vi "ATE_Bandwidth_2.vi"() -> ()   [LabVIEW 2009]
doc: "RVP8 bandwidth measuring vi - reads the primary frequency of SPOL from the ATE_settings.txt file"
uses:
  Rvp8PowerData.ctl
  <vilib>/Analysis/NI_AALBase.lvlib
  <vilib>/Analysis/NI_AALPro.lvlib
panel:
  in  "Ready":bool
  out "Instructions":string="rvp8 bandwidth measuring vi\n\nBasic operation\n1 - configure ATE switches with the yellow 'Bandwidth Setup' button\n2 - measure the bandwidth with the red 'Calibrate' button\n3 - exit the program with the red 'Exit' button\n\nHints:\nWait for the green 'READY' light before clicking buttons\nClick blue buttons after making changes on 'Controls' tab\nCheck status tab before calibration"
  out "Real Time XY":cluster{dbl[], dbl[]}(graph)
  in  "Configuration 1":bool
  out "Cal Output File":path
  out "?":cluster{dbl[], dbl[]}[](graph)
  out "RVP8 Bandwidth":cluster{dbl[], dbl[]}[](graph)
  in  "DataSource":bool
  out "File Name":string
  in  "Data Directory":string="/home/operator/ate/data/rvp8_bw"
  in  "Set SigGen":bool
  in  "Initialize":bool
  in  "70 dB":bool
  in  "121 dB":bool
  in  "Switches":bool
  in  "Calibrate":bool
  in  "Stop":bool
  in  "ATE TABS":enum32{"Status", "Controls"}(tab)=enum."Controls"
  out "ATE Switch Status":T1
  out "121dB\nAttenuators":bool[](array[boolean])
  out "70dB\nAttenuators":bool[](array[boolean])
  out "RVP8 Power":T2 {"time" format="%<%H:%M:%S\n%Y/%m/%d>T"}
  out "Signal Generator Status":T3={"Freq (GHz)"=0.0, "RF Power (dBm)"=0.0, "RF Power"=TRUE} {"Freq (GHz)" format="%.5g"; "RF Power (dBm)" format="%.2g"}
  out "121 Verified":bool
  out "70 Verfied":bool
  in  "Center Frequency (GHz)":dbl=2.809 format="%.5g"
  in  "Steps":i32=51
  in  "Steps Size (GHz)":dbl=0.0001 min=0.0 max=0.002 step=1e-06 format="%.5g"
  in  "70 dB Attn":i32=70 min=0 max=70 step=10
  in  "121 dB Attn":i32=121 min=0 max=121 step=1
  in  "ATE Switches":T4
  out "P-State":string
  out "C-State":string
  in  "Busy":bool
  # "RVP8 Bandwidth-II"
  # "1 dB"
  # "2 dB"
  # "4 dB"
  # "4 dB"
  # "10 dB"
  # "20 dB"
  # "40 dB"
  # "40 dB"
  # "10 dB"
  # "20 dB"
  # "40 dB"
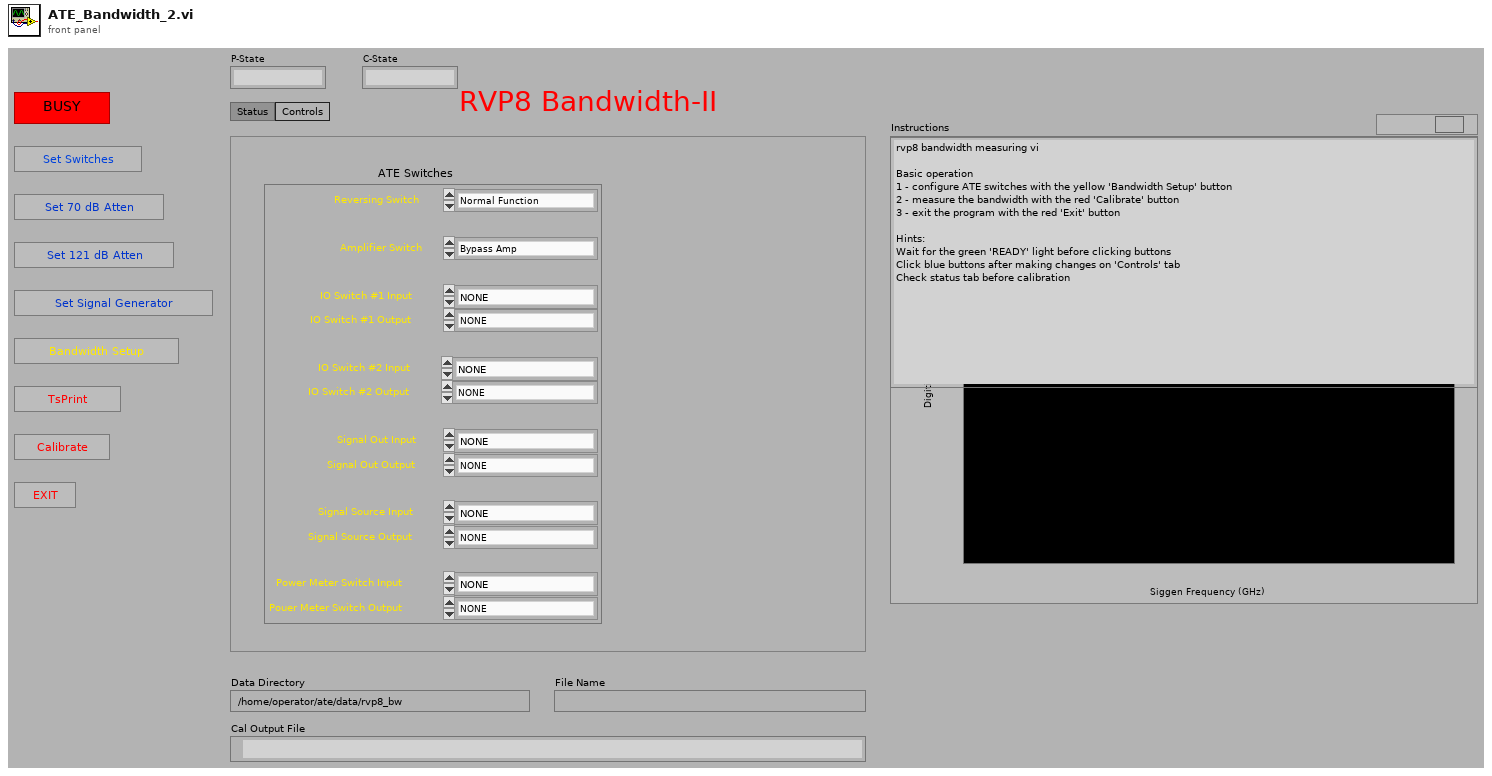
[diagram p1: front panel]
types:
  T1 = cluster{"Reversing Switch ":bool, "IO Switch #1":bool, "IO Switch #2":bool, "Signal Out":bool, "Signal Source":bool, "Power Meter":bool, "Amp By Pass":bool}
  T2 = typedef "Rvp8PowerData.ctl" = cluster{"success":bool, "time":dbl, "el":dbl, "az":dbl, "dbm0":dbl, "dbm1":dbl, "dbmHc":dbl, "dbmHx":dbl, "dbmVc":dbl, "dbmVx":dbl}
  T3 = cluster{"Freq (GHz)":dbl, "RF Power (dBm)":dbl, "RF Power":bool}
  T4 = cluster{"Reversing Switch":enum16{"Normal Function", "Reversing Function"}, "IO Switch #1 Input":enum16{"NONE", "AHR (J2)", "Splitter", "Signal Out Switch (S3)", "Reversing Switch"}, "IO Switch #1 Output":enum16{"NONE", "AHR (J2)", "Delay Device (S4)", "Power Meter Switch (S5)", "Reversing Switch"}, "IO Switch #2 Input":enum16{"NONE", "AVR (J3)", "Splitter", "Signal Out Switch (S3)", " 2W Term (TM1)", "Reversing Switch"}, "IO Switch #2 Output":enum16{"NONE", "AVR (J3)", "Signal Out Switch (S3)", "Power Meter Switch (S5)", "Reversing Switch", "2W Term (TM1)"}, "Signal Out Input":enum16{"NONE", "Amp Bypass Switch (S6)", "IO Switch #1 (S1)", "IO Switch #2 (S2)", "2W Term (TM3)"}, "Signal Out Output":enum16{"NONE", "2 Watt Term (TM3)", "Splitter", "Power Meter Switch (S5)"}, "Signal Source Input":enum16{"NONE", "Delay Device", "Signal Generator (J7)", "Inside Noise Box NF (J5)", "2W Term (TM3)"}, "Signal Source Output":enum16{"NONE", "Amp Bypass Switch", "Test Pulse Generator", "Power Meter Switch (S5)"}, "Power Meter Switch Input":enum16{"NONE", "IO Switch #1 (S1)", "Signal Source Switch (S4)", "Signal Out Switch (S3)", "IO Switch #2 (S2)", "TXH-TXV Switch (J8)"}, "Pouer Meter Switch Output":enum16{"NONE", "Power Meter (J6)"}, "Amplifier Switch":enum16{"Bypass Amp", "Include Amp"}}
  T5 = cluster{"Frequency (GHz)":dbl, "RF Power (dBm)":dbl, "RF ON/OFF":bool}
  T6 = enum16{"open", "replace", "create", "open or create", "replace or create", "replace or create with confirmation"}
  T7 = cluster{"Frequency (GHz)":dbl, "RF Power (dBm)":dbl, "RF Power":bool}
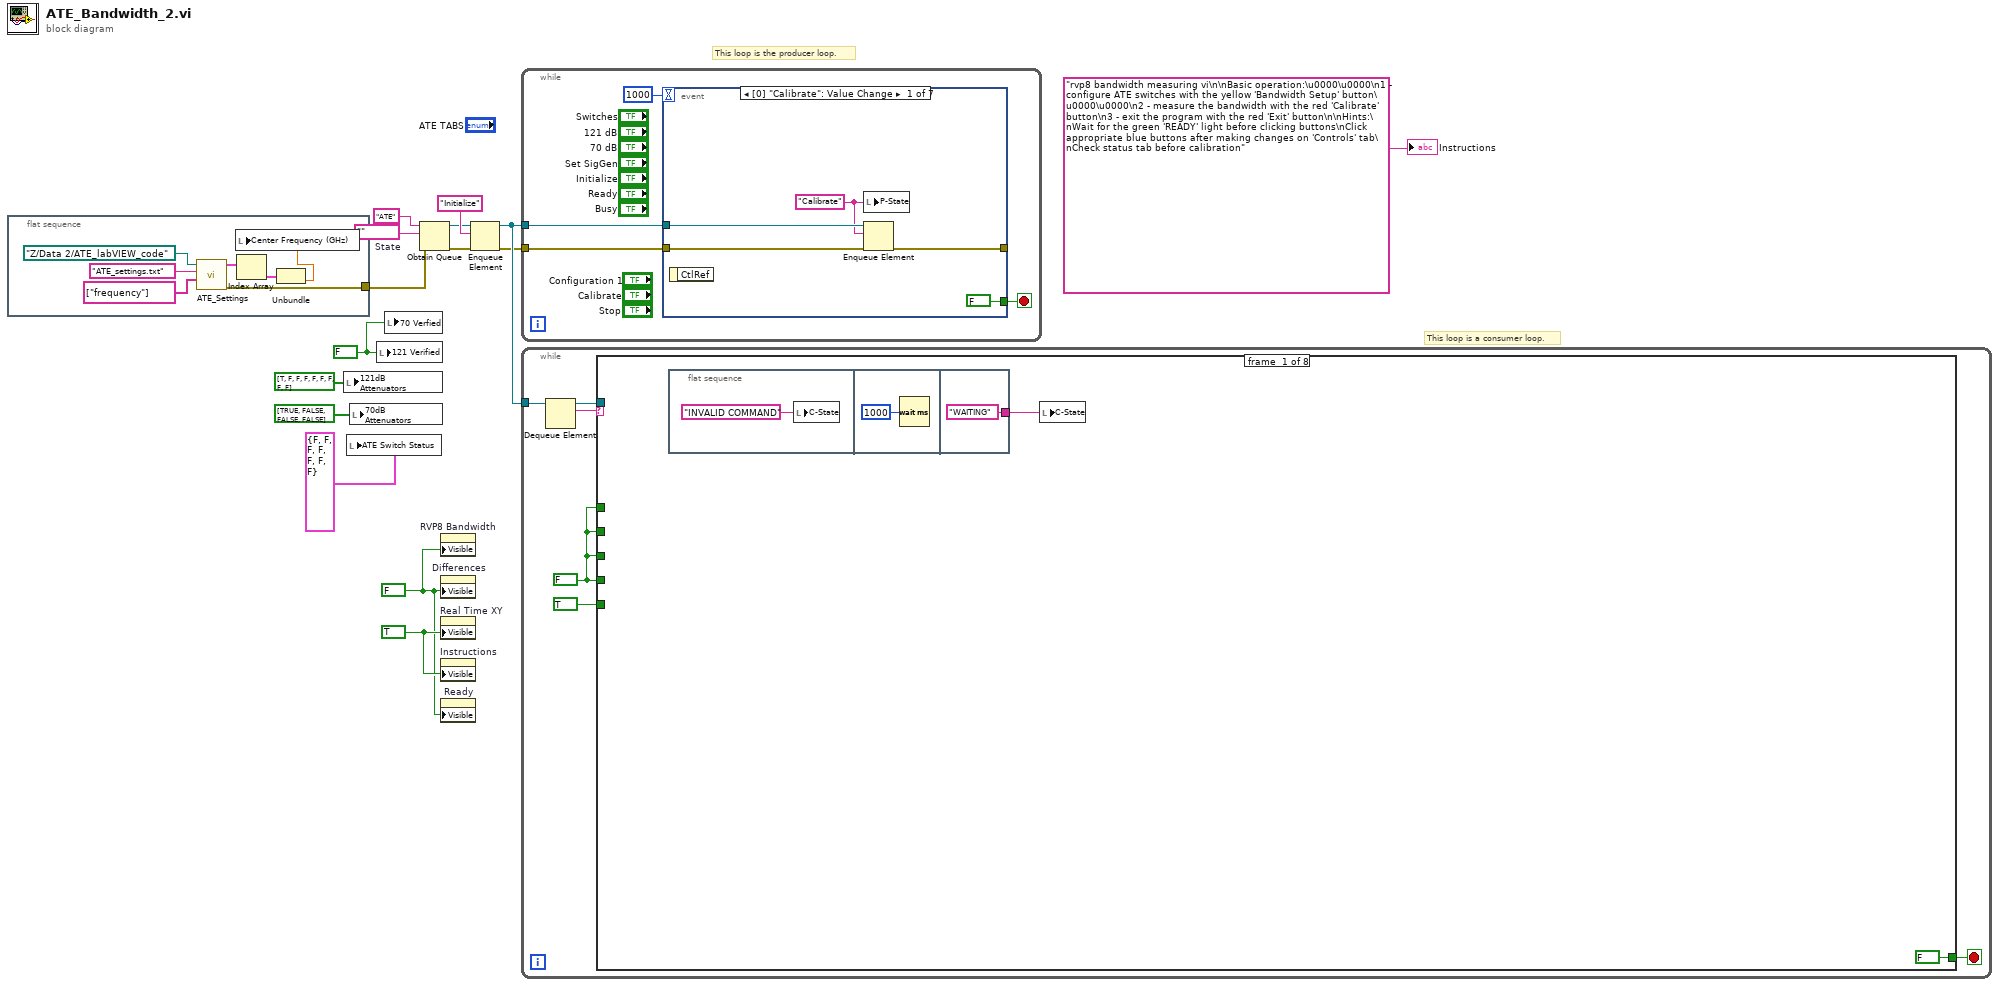
[diagram p0: block diagram]
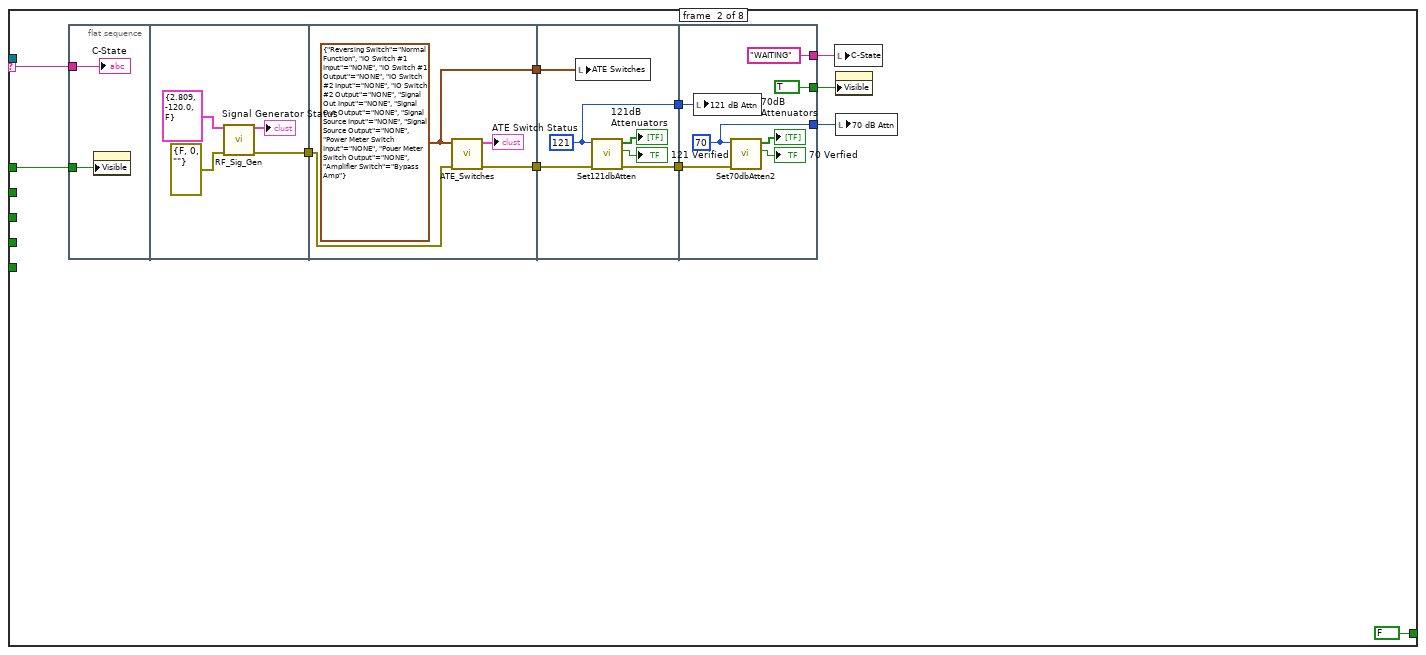
[diagram p2: hidden frame]
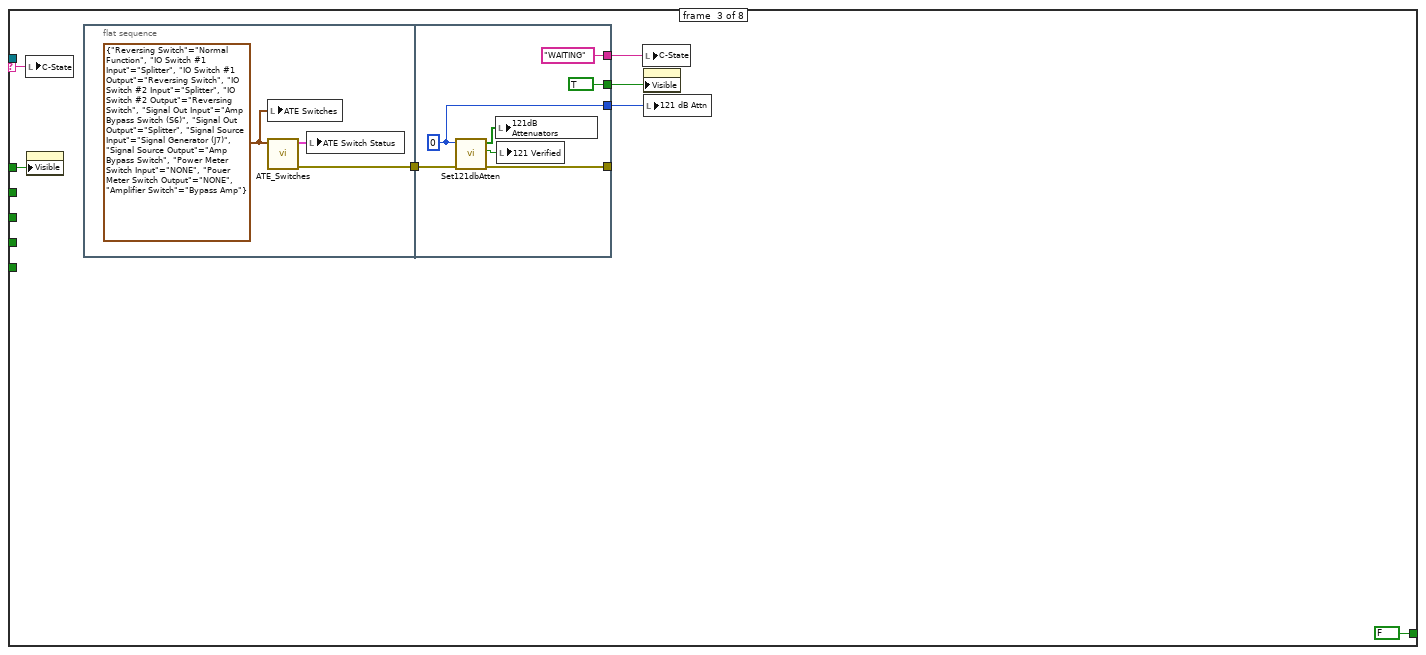
[diagram p3: hidden frame]
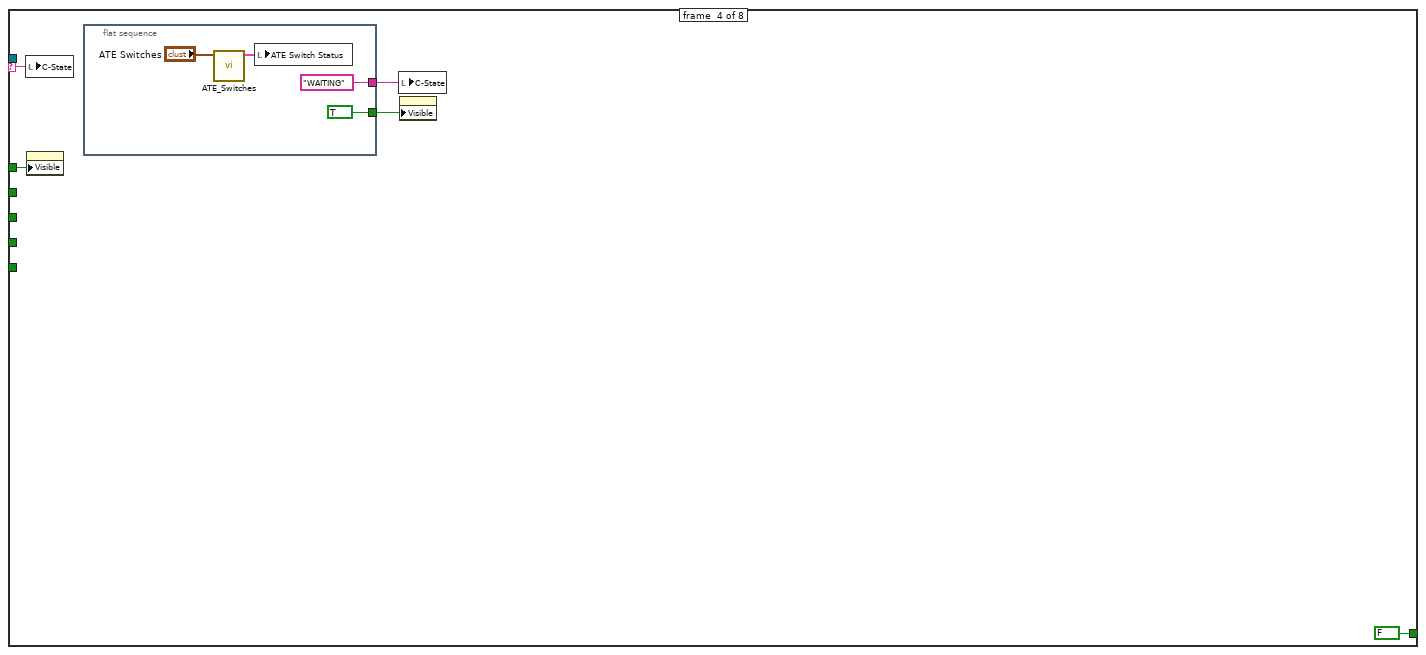
[diagram p4: hidden frame]
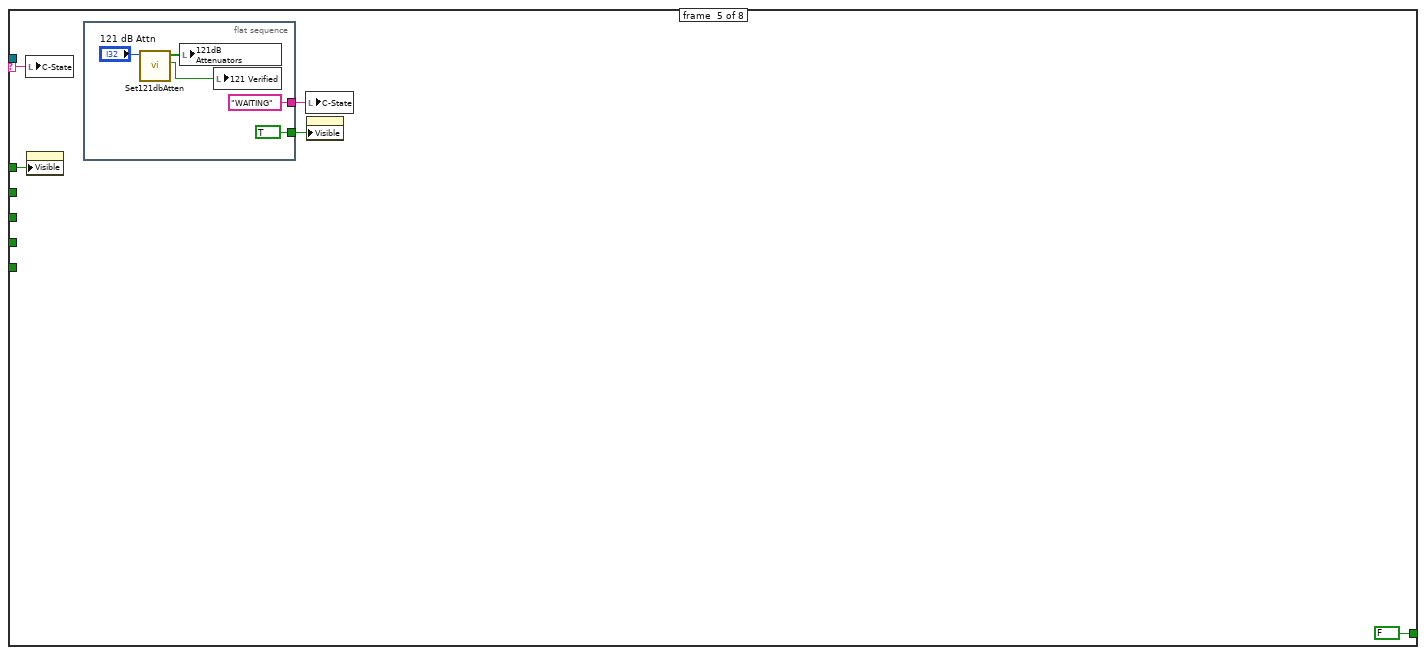
[diagram p5: hidden frame]
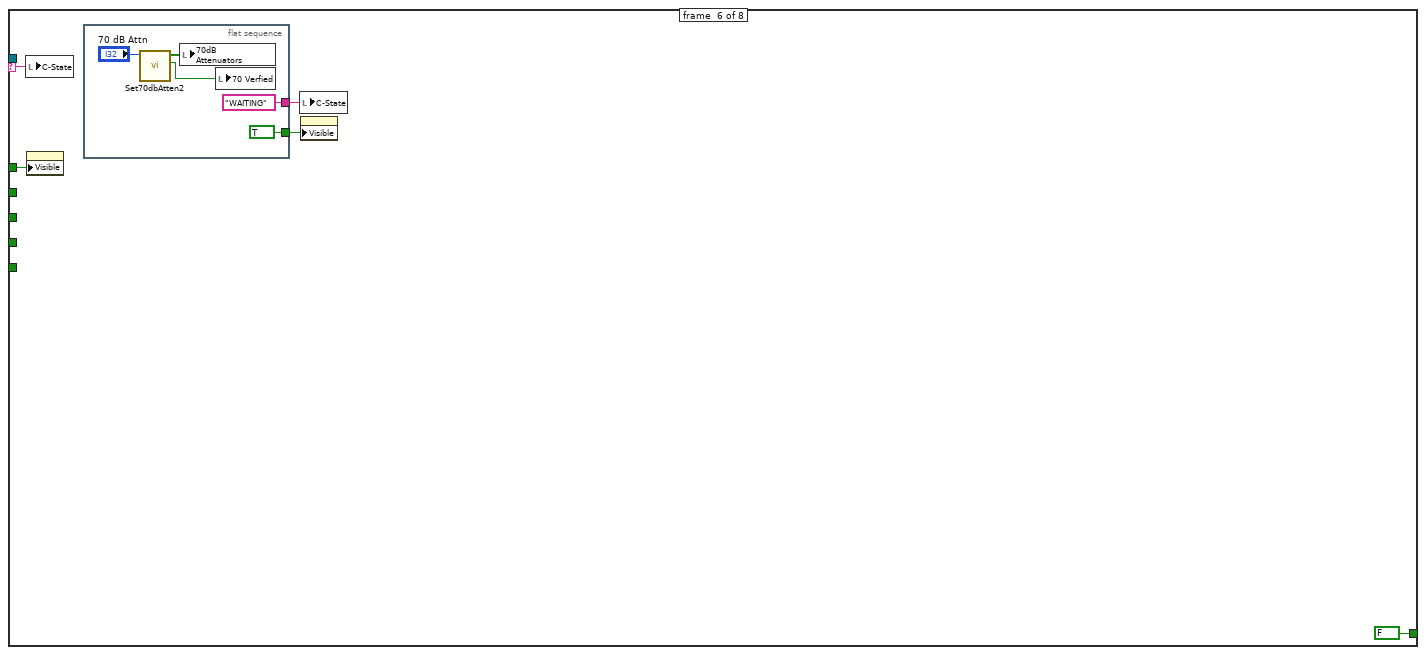
[diagram p6: hidden frame]
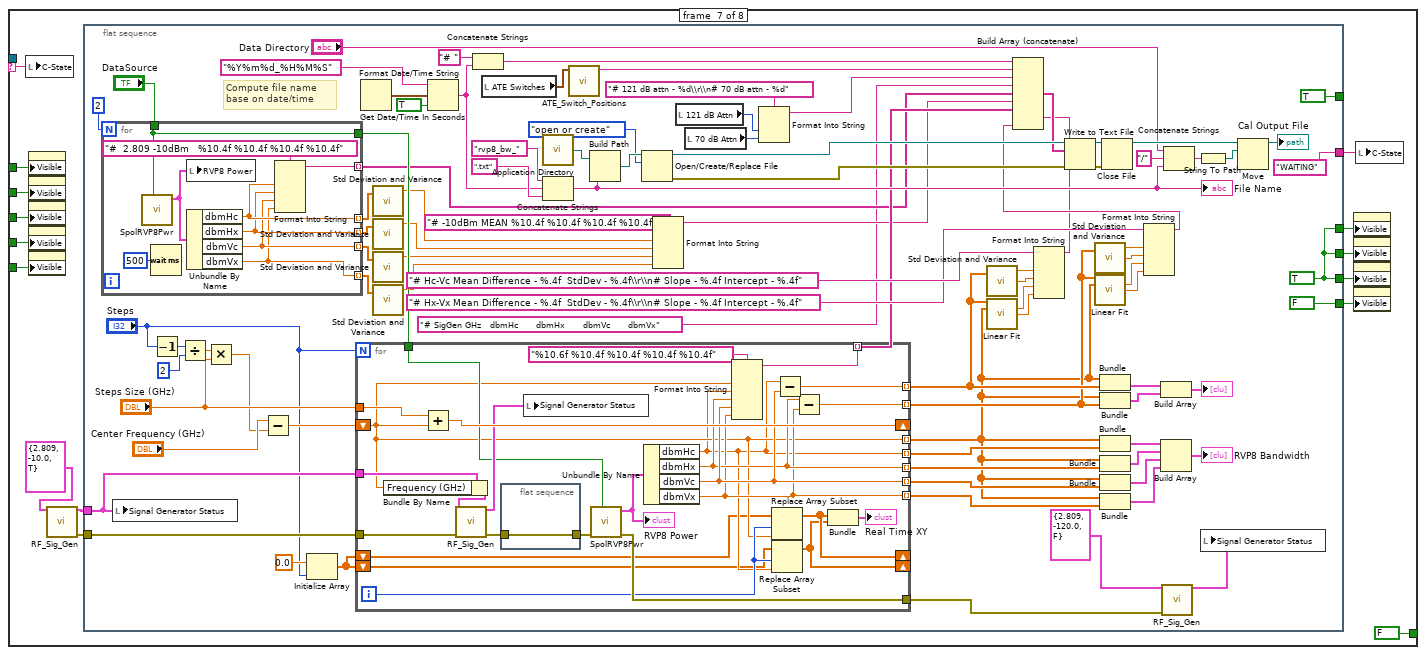
[diagram p7: hidden frame]
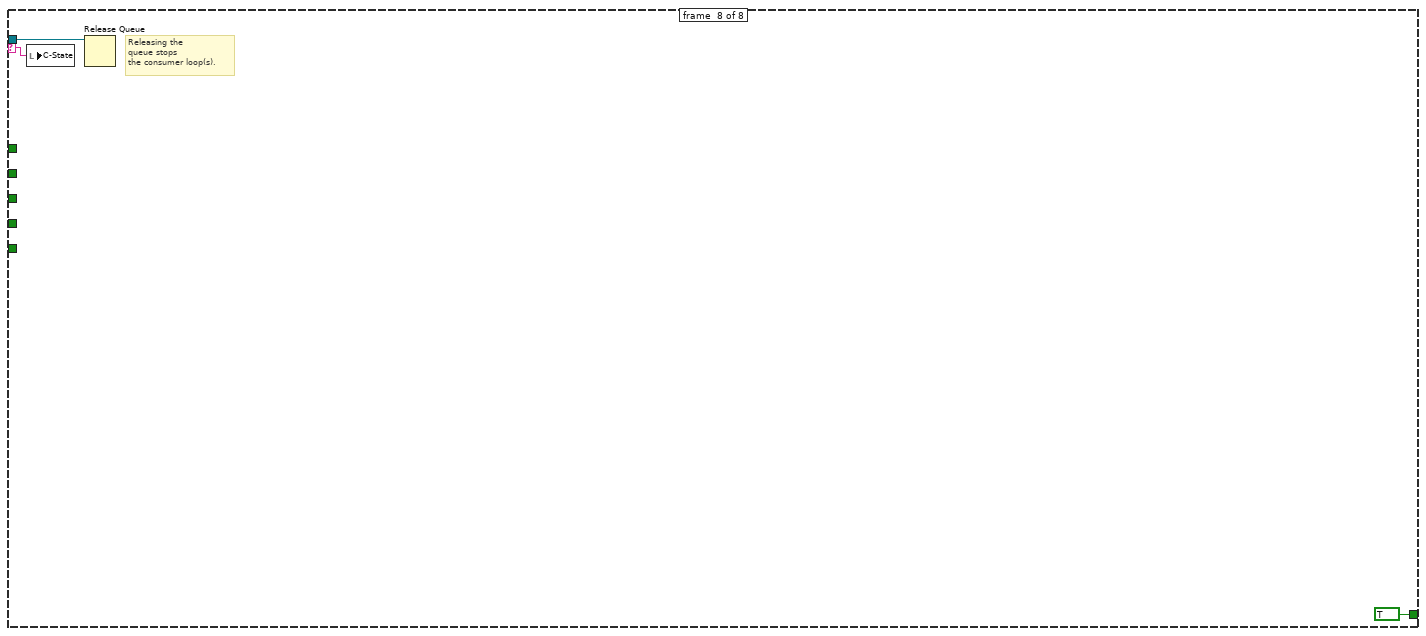
[diagram p8: hidden frame]
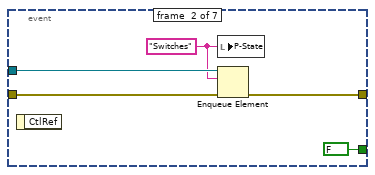
[diagram p9: hidden frame]
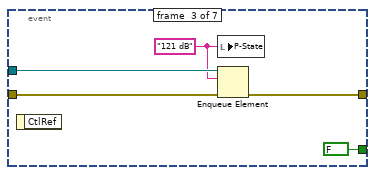
[diagram p10: hidden frame]
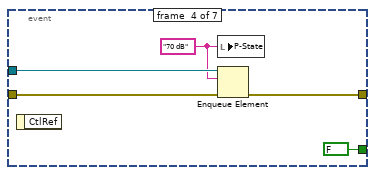
[diagram p11: hidden frame]
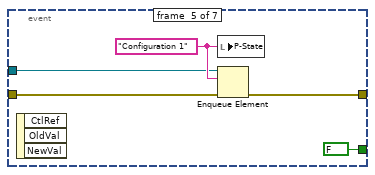
[diagram p12: hidden frame]
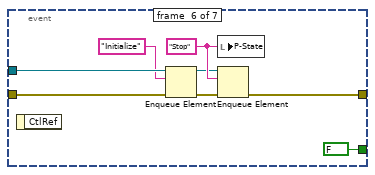
[diagram p13: hidden frame]
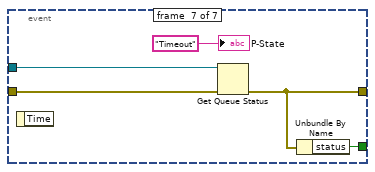
[diagram p14: hidden frame]
diagram:
  w2 = FALSE ("Visible")
  w3 = TRUE ("Visible")
  w5 = FALSE ("70 Verfied")
  w15 = ""  # State
  # "This loop is the producer loop."
  # "This loop is a consumer loop."
  n1 = flat-sequence {
    tunnel: [w22] -> w1
    frame #0 {
      n2 = call "ATE_Settings.vi"("Variable to Read"=string[] ["frequency"], "file name"="ATE_settings.txt", "start path"=path "Z:/Data 2/ATE_labVIEW_code") -> ("error out"=w22:errorcluster, "NewVariables"=w18:cluster{"Name":string, "Value":dbl}[])  [unwired: 7 in]
      n3 = Index Array(array=w18) -> (element=w17:cluster{"Name":string, "Value":dbl})  [unwired: 1 in]
      n4 = Unbundle(w17) -> ("Value"=w16:dbl)  [unwired: 1 out]
      n5 = local write "Center Frequency (GHz)"(w16) -> ()
    }
  }
  n6 = local write "121dB\nAttenuators"(bool[] [TRUE, FALSE, FALSE, FALSE, FALSE, FALSE, FALSE, FALSE, FALSE] ("121dB\nAttenuators")) -> ()
  n7 = local write "ATE Switch Status"(T1 {"Reversing Switch "=FALSE, "IO Switch #1"=FALSE, "IO Switch #2"=FALSE, "Signal Out"=FALSE, "Signal Source"=FALSE, "Power Meter"=FALSE, "Amp By Pass"=FALSE} ("ATE Switch Status")) -> ()
  n8 = local write "70dB\nAttenuators"(bool[] [TRUE, FALSE, FALSE, FALSE] ("70dB\nAttenuators")) -> ()
  n9 = local write "121 Verified"(w5) -> ()
  n10 = local write "70 Verfied"(w5) -> ()
  n11 = Obtain Queue(name (unnamed)="ATE", element data type=w15, error in (no error)=w1) -> (queue out=w12:refnum<queue>, error out=w10:errorcluster)  [unwired: 2 in, 1 out]
  n12 = property on="RVP8 Bandwidth" class="XYGraph (strict)"("Visible"=w2) -> ()  [unwired: 2 in, 2 out]
  n13 = property on="Differences" class="XYGraph (strict)"("Visible"=w2) -> ()  [unwired: 2 in, 2 out]
  n14 = property on="Real Time XY" class="XYGraph (strict)"("Visible"=w3) -> ()  [unwired: 2 in, 2 out]
  n15 = property on="Instructions" class="Str"("Visible"=w3) -> ()  [unwired: 2 in, 2 out]
  n16 = property on="Ready" class="Bool"("Visible"=w2) -> ()  [unwired: 2 in, 2 out]
  n17 = Enqueue Element(queue=w12, element="Initialize", error in (no error)=w10) -> (queue out=w11:refnum<queue>, error out=w9:errorcluster)  [unwired: 1 in, 1 out]
  n18 = while {
    tunnel: w11 -> [w26]
    tunnel: w9 -> [w25]
    stop <- w23 stop-if-true
    n19 = event shown="[0] \"Calibrate\": Value Change" {
      selector: _ -> [_ _ _ _ _ _ _]
      dyn-events: _ -> [_ _ _ _ _ _ _]
      timeout: 1000 -> [_ _ _ _ _ _ _]
      tunnel: w26 -> [w31 w36 w41 w46 w50 w54 w64]
      tunnel: w25 -> [w30 w35 w40 w45 w49 w56 w60]
      tunnel: [w29 w34 w39 w44 w48 w59 w62] -> _
      tunnel: [FALSE FALSE FALSE FALSE FALSE ("status") FALSE w63] -> w23
      event #0 {
        w27 = "Calibrate" ("element")
        n20 = event-data() -> ()  [unwired: 1 in, 1 out]
        n21 = local write "P-State"(w27) -> ()
        n22 = Enqueue Element(queue=w31, element=w27, error in (no error)=w30) -> (error out=w29:errorcluster)  [unwired: 1 in, 2 out]
      }
      event #1 {
        w32 = "Switches" ("element")
        n23 = event-data() -> ()  [unwired: 1 in, 1 out]
        n24 = local write "P-State"(w32) -> ()
        n25 = Enqueue Element(queue=w36, element=w32, error in (no error)=w35) -> (error out=w34:errorcluster)  [unwired: 1 in, 2 out]
      }
      event #2 {
        w37 = "121 dB" ("element")
        n26 = event-data() -> ()  [unwired: 1 in, 1 out]
        n27 = local write "P-State"(w37) -> ()
        n28 = Enqueue Element(queue=w41, element=w37, error in (no error)=w40) -> (error out=w39:errorcluster)  [unwired: 1 in, 2 out]
      }
      event #3 {
        w42 = "70 dB" ("element")
        n29 = event-data() -> ()  [unwired: 1 in, 1 out]
        n30 = local write "P-State"(w42) -> ()
        n31 = Enqueue Element(queue=w46, element=w42, error in (no error)=w45) -> (error out=w44:errorcluster)  [unwired: 1 in, 2 out]
      }
      event #4 {
        w51 = "Configuration 1" ("element")
        n32 = event-data() -> ()  [unwired: 1 in, 3 out]
        n33 = local write "P-State"(w51) -> ()
        n34 = Enqueue Element(queue=w50, element=w51, error in (no error)=w49) -> (error out=w48:errorcluster)  [unwired: 1 in, 2 out]
      }
      event #5 {
        w57 = "Stop" ("element")
        n35 = event-data() -> ()  [unwired: 1 in, 1 out]
        n36 = Enqueue Element(queue=w54, element="Initialize", error in (no error)=w56) -> (queue out=w53:refnum<queue>, error out=w55:errorcluster)  [unwired: 1 in, 1 out]
        n37 = local write "P-State"(w57) -> ()
        n38 = Enqueue Element(queue=w53, element=w57, error in (no error)=w55) -> (error out=w59:errorcluster)  [unwired: 1 in, 2 out]
      }
      event #6 {
        n39 = event-data() -> ()  [unwired: 1 in, 1 out]
        n40 = Get Queue Status(queue=w64, error in (no error)=w60) -> (error out=w62:errorcluster)  [unwired: 1 in, 7 out]
        n41 = Unbundle By Name(w62) -> ("status"=w63:bool)
        "P-State" <- "Timeout" ("element")
      }
    }
  }
  n42 = while {
    tunnel: w11 -> [w70]
    stop <- w67 stop-if-true
    w65 = FALSE ("Visible")
    n43 = Dequeue Element(queue=w70) -> (queue out=w68:refnum<queue>, element=w69:string)  [unwired: 2 in, 2 out]
    n44 = case shown="\"Initialize\"" w69 {
      selector: w69 -> [_ w76 w112 w131 w139 w149 w169 w299]
      tunnel: w68 -> [_ _ _ _ _ _ _ w298]
      tunnel: [FALSE FALSE FALSE FALSE FALSE FALSE FALSE TRUE] -> w67
      tunnel: w65 -> [_ _ _ _ _ _ w164 _]
      tunnel: w65 -> [_ _ _ _ _ _ w163 _]
      tunnel: TRUE ("Visible") -> [_ _ _ _ _ _ w162 _]
      tunnel: w65 -> [_ _ _ _ _ _ w158 _]
      tunnel: w65 -> [_ w77 w111 w128 w137 w147 w157 _]
      frame #0 {
        n45 = flat-sequence {
          tunnel: ["WAITING" ("element")] -> w71
          frame #0 {
            n46 = local write "C-State"("INVALID COMMAND" ("C-State")) -> ()
          }
          frame #1 {
            n47 = Wait (ms)(milliseconds to wait=u32 1000) -> ()  [unwired: 1 out]
          }
          frame #2 {
          }
        }
        n48 = local write "C-State"(w71) -> ()
      }
      frame #1 {
        n49 = flat-sequence {
          tunnel: w77 -> [w88]
          tunnel: w76 -> [w87]
          tunnel: [w89] -> w80
          tunnel: [w94] -> w83
          tunnel: w80 -> [w95]
          tunnel: [w93] -> w79
          tunnel: w83 -> [w101]
          tunnel: [w100] -> w84
          tunnel: [w99] -> w82
          tunnel: w79 -> [w97]
          tunnel: ["WAITING" ("element")] -> w85
          tunnel: w84 -> [w108]
          tunnel: w82 -> [w106]
          tunnel: [w105] -> w81
          tunnel: [TRUE ("Visible")] -> w78
          frame #0 {
            n50 = property on="Ready" class="Bool"("Visible"=w88) -> ()  [unwired: 2 in, 2 out]
            "C-State" <- w87
          }
          frame #1 {
            n51 = call "RF_Sig_Gen.vi"("Signal Generator Control"=T5 {"Frequency (GHz)"=2.809, "RF Power (dBm)"=-120.0, "RF ON/OFF"=FALSE}, "error in"=errorcluster {"status"=FALSE, "code"=0, "source"=""}) -> ("Signal Generator Status"=→"Signal Generator Status":T7, "Sig Gen Errors"=w89:errorcluster)  [unwired: 12 in]
          }
          frame #2 {
            w93 = T4 {"Reversing Switch"=enum."Normal Function", "IO Switch #1 Input"=enum."NONE", "IO Switch #1 Output"=enum."NONE", "IO Switch #2 Input"=enum."NONE", "IO Switch #2 Output"=enum."NONE", "Signal Out Input"=enum."NONE", "Signal Out Output"=enum."NONE", "Signal Source Input"=enum."NONE", "Signal Source Output"=enum."NONE", "Power Meter Switch Input"=enum."NONE", "Pouer Meter Switch Output"=enum."NONE", "Amplifier Switch"=enum."Bypass Amp"} ("ATE Switches")
            n52 = call "ATE_Switches.vi"("error in"=w95, "ATE Switches"=w93) -> ("Switch Errors"=w94:errorcluster, "ATE Switch Status"=→"ATE Switch Status":T1)  [unwired: 8 in]
          }
          frame #3 {
            w99 = 121 ("Attenuation (dB)")
            n53 = local write "ATE Switches"(w97) -> ()
            n54 = call "Set121dbAtten.vi"("error in (no error)"=w101, "Attenuation (dB)"=w99) -> ("error out"=w100:errorcluster, "Verfied"=→"121 Verified":bool, "Active Attenuators"=→"121dB\nAttenuators":bool[])  [unwired: 7 in]
          }
          frame #4 {
            w105 = 70 ("Attenuation (dB)")
            n55 = local write "121 dB Attn"(w106) -> ()
            n56 = call "Set70dbAtten2.vi"("error in (no error)"=w108, "Attenuation (dB)"=w105) -> ("Verfied"=→"70 Verfied":bool, "Active Attenuators"=→"70dB\nAttenuators":bool[])  [unwired: 7 in, 1 out]
          }
        }
        n57 = local write "C-State"(w85) -> ()
        n58 = property on="Ready" class="Bool"("Visible"=w78) -> ()  [unwired: 2 in, 2 out]
        n59 = local write "70 dB Attn"(w81) -> ()
      }
      frame #2 {
        n60 = local write "C-State"(w112) -> ()
        n61 = property on="Ready" class="Bool"("Visible"=w111) -> ()  [unwired: 2 in, 2 out]
        n62 = flat-sequence {
          tunnel: [w119] -> w115
          tunnel: w115 -> [w126]
          tunnel: [w121] -> w114
          tunnel: ["WAITING" ("element")] -> w113
          tunnel: [w124] -> _
          tunnel: [TRUE ("Visible")] -> w110
          frame #0 {
            w117 = T4 {"Reversing Switch"=enum."Normal Function", "IO Switch #1 Input"=enum."Splitter", "IO Switch #1 Output"=enum."Reversing Switch", "IO Switch #2 Input"=enum."Splitter", "IO Switch #2 Output"=enum."Reversing Switch", "Signal Out Input"=enum."Amp Bypass Switch (S6)", "Signal Out Output"=enum."Splitter", "Signal Source Input"=enum."Signal Generator (J7)", "Signal Source Output"=enum."Amp Bypass Switch", "Power Meter Switch Input"=enum."NONE", "Pouer Meter Switch Output"=enum."NONE", "Amplifier Switch"=enum."Bypass Amp"} ("ATE Switches")
            n63 = local write "ATE Switches"(w117) -> ()
            n64 = call "ATE_Switches.vi"("ATE Switches"=w117) -> ("Switch Errors"=w119:errorcluster, "ATE Switch Status"=w118:T1)  [unwired: 9 in]
            n65 = local write "ATE Switch Status"(w118) -> ()
          }
          frame #1 {
            w121 = 0 ("Attenuation (dB)")
            n66 = call "Set121dbAtten.vi"("error in (no error)"=w126, "Attenuation (dB)"=w121) -> ("error out"=w124:errorcluster, "Verfied"=w122:bool, "Active Attenuators"=w123:bool[])  [unwired: 7 in]
            n67 = local write "121dB\nAttenuators"(w123) -> ()
            n68 = local write "121 Verified"(w122) -> ()
          }
        }
        n69 = local write "C-State"(w113) -> ()
        n70 = property on="Ready" class="Bool"("Visible"=w110) -> ()  [unwired: 2 in, 2 out]
        n71 = local write "121 dB Attn"(w114) -> ()
      }
      frame #3 {
        n72 = local write "C-State"(w131) -> ()
        n73 = property on="Ready" class="Bool"("Visible"=w128) -> ()  [unwired: 2 in, 2 out]
        n74 = flat-sequence {
          tunnel: ["WAITING" ("element")] -> w129
          tunnel: [TRUE ("Visible")] -> w127
          frame #0 {
            n75 = call "ATE_Switches.vi"("ATE Switches"="ATE Switches") -> ("ATE Switch Status"=w134:T1)  [unwired: 9 in, 1 out]
            n76 = local write "ATE Switch Status"(w134) -> ()
          }
        }
        n77 = local write "C-State"(w129) -> ()
        n78 = property on="Ready" class="Bool"("Visible"=w127) -> ()  [unwired: 2 in, 2 out]
      }
      frame #4 {
        n79 = local write "C-State"(w139) -> ()
        n80 = property on="Ready" class="Bool"("Visible"=w137) -> ()  [unwired: 2 in, 2 out]
        n81 = flat-sequence {
          tunnel: ["WAITING" ("element")] -> w138
          tunnel: [TRUE ("Visible")] -> w136
          frame #0 {
            n82 = call "Set121dbAtten.vi"("Attenuation (dB)"="121 dB Attn") -> ("Verfied"=w143:bool, "Active Attenuators"=w145:bool[])  [unwired: 8 in, 1 out]
            n83 = local write "121dB\nAttenuators"(w145) -> ()
            n84 = local write "121 Verified"(w143) -> ()
          }
        }
        n85 = local write "C-State"(w138) -> ()
        n86 = property on="Ready" class="Bool"("Visible"=w136) -> ()  [unwired: 2 in, 2 out]
      }
      frame #5 {
        n87 = local write "C-State"(w149) -> ()
        n88 = property on="Ready" class="Bool"("Visible"=w147) -> ()  [unwired: 2 in, 2 out]
        n89 = flat-sequence {
          tunnel: ["WAITING" ("element")] -> w148
          tunnel: [TRUE ("Visible")] -> w146
          frame #0 {
            n90 = call "Set70dbAtten2.vi"("Attenuation (dB)"="70 dB Attn") -> ("Verfied"=w152:bool, "Active Attenuators"=w154:bool[])  [unwired: 8 in, 1 out]
            n91 = local write "70dB\nAttenuators"(w154) -> ()
            n92 = local write "70 Verfied"(w152) -> ()
          }
        }
        n93 = local write "C-State"(w148) -> ()
        n94 = property on="Ready" class="Bool"("Visible"=w146) -> ()  [unwired: 2 in, 2 out]
      }
      frame #6 {
        n95 = local write "C-State"(w169) -> ()
        n96 = property on="Ready" class="Bool"("Visible"=w157) -> ()  [unwired: 2 in, 2 out]
        n97 = property on="Instructions" class="Str"("Visible"=w158) -> ()  [unwired: 2 in, 2 out]
        n98 = property on="RVP8 Bandwidth" class="XYGraph (strict)"("Visible"=w164) -> ()  [unwired: 2 in, 2 out]
        n99 = property class="XYGraph (strict)"("Visible"=w163) -> ()  [unwired: 2 in, 2 out]
        n100 = property on="Real Time XY" class="XYGraph (strict)"("Visible"=w162) -> ()  [unwired: 2 in, 2 out]
        n101 = call "RF_Sig_Gen.vi"("Signal Generator Control"=T5 {"Frequency (GHz)"=2.809, "RF Power (dBm)"=-10.0, "RF ON/OFF"=TRUE}) -> ("Signal Generator Status"=w167:T7, "Sig Gen Errors"=w166:errorcluster)  [unwired: 13 in]
        n102 = flat-sequence {
          tunnel: ["WAITING" ("element")] -> w168
          tunnel: w167 -> [w182]
          tunnel: w166 -> [w183]
          tunnel: [w171] -> w161
          tunnel: [w171] -> w160
          tunnel: [FALSE ("Visible")] -> w159
          tunnel: [TRUE ("Visible")] -> _
          tunnel: [w171] -> w156
          frame #0 {
            w171 = TRUE ("Visible")
            # "Compute file name base on date/time"
            n103 = for {
              N: 2 -> [_]
              tunnel: [w268] -> w187 mode=indexing
              tunnel: [w267] -> w200 mode=indexing
              tunnel: [w266] -> w201 mode=indexing
              tunnel: [w265] -> w202 mode=indexing
              tunnel: [w262] -> w203 mode=indexing
              tunnel: "DataSource" -> [w264]
              tunnel: [w264] -> w197
              n104 = call "SpolRVP8Pwr.vi"("DataSource"=w264) -> ("RVP8_power"=w263:T2)  [unwired: 7 in, 3 out]
              n105 = Wait (ms)(milliseconds to wait=u32 500) -> ()  [unwired: 1 out]
              n106 = local write "RVP8 Power"(w263) -> ()
              n107 = Unbundle By Name(w263) -> ("dbmHc"=w267:dbl, "dbmHx"=w266:dbl, "dbmVc"=w265:dbl, "dbmVx"=w262:dbl)
              n108 = Format Into String(format string="#  2.809 -10dBm   %10.4f %10.4f %10.4f %10.4f", w267, w266, w265, w262) -> (resulting string=w268:string)  [unwired: 2 in, 1 out]
            }
            n109 = local write "Signal Generator Status"(w182) -> ()
            n110 = Decrement(x="Steps") -> (x-1=w185:i32)
            n111 = Divide(x=w185, y=2) -> (x/y=w181:dbl)
            n112 = Multiply(x=w181, y="Steps Size (GHz)") -> (x*y=w177:dbl)
            n113 = Subtract(x="Center Frequency (GHz)", y=w177) -> (x-y=w180:dbl)
            n114 = Initialize Array(0.0 ("element"), "Steps") -> (w174:dbl[])
            n115 = for {
              N: "Steps" -> [_]
              shift-right: [w285] -> _
              shift-left: w180 -> [w276]
              tunnel: w183 -> [w293]
              tunnel: [w276] -> w218 mode=indexing
              tunnel: [w275] -> w254 mode=indexing
              tunnel: [w283] -> w253 mode=indexing
              tunnel: [w284] -> w252 mode=indexing
              tunnel: [w282] -> w251 mode=indexing
              tunnel: [w296] -> w189 mode=indexing
              tunnel: [w287] -> w220 mode=indexing
              tunnel: [w286] -> w219 mode=indexing
              tunnel: w182 -> [w294]
              tunnel: [w290] -> w231
              tunnel: w197 -> [w280]
              tunnel: "Steps Size (GHz)" -> [w279]
              shift-right: [w272] -> _
              shift-left: w174 -> [w273]
              shift-right: [w271] -> _
              shift-left: w174 -> [w274]
              i -> [w277]
              n116 = Bundle By Name(cluster=w294, "Frequency (GHz)"=w276) -> (w288:T7)
              n117 = Add(x=w279, y=w276) -> (x+y=w285:dbl)
              n118 = call "RF_Sig_Gen.vi"("Signal Generator Control"=w288, "error in"=w293) -> ("Signal Generator Status"=w281:T7, "Sig Gen Errors"=w292:errorcluster)  [unwired: 12 in]
              n119 = flat-sequence {
                tunnel: w292 -> [w297]
                tunnel: [w297] -> w291
                frame #0 {
                }
              }
              n120 = local write "Signal Generator Status"(w281) -> ()
              n121 = call "SpolRVP8Pwr.vi"("DataSource"=w280, "error in (no error)"=w291) -> ("Comm error"=w290:errorcluster, "RVP8_power"=w295:T2)  [unwired: 6 in, 2 out]
              "RVP8 Power" <- w295
              n122 = Unbundle By Name(w295) -> ("dbmHc"=w275:dbl, "dbmHx"=w283:dbl, "dbmVc"=w284:dbl, "dbmVx"=w282:dbl)
              n123 = Format Into String(format string="%10.6f %10.4f %10.4f %10.4f %10.4f", w276, w275, w283, w284, w282) -> (resulting string=w296:string)  [unwired: 2 in, 1 out]
              n124 = Replace Array Subset(array=w273, new element=w276, index=w277) -> (w272:dbl[])
              n125 = Replace Array Subset(array=w274, new element=w275, index=w277) -> (w271:dbl[])
              n126 = Subtract(x=w275, y=w284) -> (x-y=w287:dbl)
              n127 = Subtract(x=w283, y=w282) -> (x-y=w286:dbl)
              n128 = Bundle(w272, w271) -> (→"Real Time XY":cluster{dbl[], dbl[]})  [unwired: 1 in]
            }
            n129 = Get Date/Time In Seconds() -> (seconds since 1Jan1904=w256:timestamp)
            n130 = call <vilib>:"Std Deviation and Variance.vi"("X"=w200) -> ("mean"=w194:dbl)  [unwired: 1 in, 2 out]
            n131 = call <vilib>:"Std Deviation and Variance.vi"("X"=w201) -> ("mean"=w193:dbl)  [unwired: 1 in, 2 out]
            n132 = call <vilib>:"Std Deviation and Variance.vi"("X"=w202) -> ("mean"=w192:dbl)  [unwired: 1 in, 2 out]
            n133 = call <vilib>:"Std Deviation and Variance.vi"("X"=w203) -> ("mean"=w195:dbl)  [unwired: 1 in, 2 out]
            n134 = Format Date/Time String(time format string (%c)="%Y%m%d_%H%M%S", seconds (now)=w256, UTC format=TRUE) -> (date/time string=w210:string)
            n135 = Concatenate Strings("# " ("string"), w210) -> (w209:string)
            n136 = local read "ATE Switches"() -> (w229:T4)
            n137 = call <vilib>:"Application Directory.vi"() -> ("Application Directory"=w255:path)
            n138 = Concatenate Strings("rvp8_bw_", w210, ".txt") -> (w206:string)
            "File Name" <- w206
            n139 = call "ATE_Switch_Positions.vi"("ATE Switches"=w229) -> ("ATE Switch/Position"=w208:string)  [unwired: 10 in]
            n140 = Build Path(base path=w255, name or relative path=w206) -> (appended path=w242:path)
            n141 = Open/Create/Replace File(file path (use dialog)=w242, operation (0:open)=T6."open or create") -> (refnum out=w241:refnum<file>, error out=w240:errorcluster)  [unwired: 4 in, 1 out]
            n142 = Format Into String(format string="# -10dBm MEAN %10.4f %10.4f %10.4f %10.4f", w194, w193, w192, w195) -> (resulting string=w188:string)  [unwired: 2 in, 1 out]
            n143 = local read "121 dB Attn"() -> (w226:i32)
            n144 = local read "70 dB Attn"() -> (w225:i32)
            n145 = Format Into String(format string="# 121 dB attn - %d\\r\\n# 70 dB attn - %d", w226, w225) -> (resulting string=w207:string)  [unwired: 2 in, 1 out]
            n146 = call <vilib>:"Std Deviation and Variance.vi"("X"=w220) -> ("mean"=w224:dbl, "standard deviation"=w221:dbl)  [unwired: 1 in, 1 out]
            n147 = call <vilib>:"Linear Fit.vi"("Y"=w220, "X"=w218) -> ("slope"=w223:dbl, "intercept"=w222:dbl)  [unwired: 9 in, 3 out]
            n148 = Format Into String(format string="# Hc-Vc Mean Difference - %.4f  StdDev - %.4f\\r\\n# Slope - %.4f Intercept - %.4f", w224, w221, w223, w222) -> (resulting string=w190:string)  [unwired: 2 in, 1 out]
            n149 = call <vilib>:"Std Deviation and Variance.vi"("X"=w219) -> ("mean"=w217:dbl, "standard deviation"=w216:dbl)  [unwired: 1 in, 1 out]
            n150 = call <vilib>:"Linear Fit.vi"("Y"=w219, "X"=w218) -> ("slope"=w215:dbl, "intercept"=w214:dbl)  [unwired: 9 in, 3 out]
            n151 = Bundle(w218, w220) -> (w250:cluster{dbl[], dbl[]})  [unwired: 1 in]
            n152 = Bundle(w218, w219) -> (w249:cluster{dbl[], dbl[]})  [unwired: 1 in]
            n153 = Bundle(w218, w254) -> (w248:cluster{dbl[], dbl[]})  [unwired: 1 in]
            n154 = Bundle(w218, w253) -> (w247:cluster{dbl[], dbl[]})  [unwired: 1 in]
            n155 = Bundle(w218, w252) -> (w245:cluster{dbl[], dbl[]})  [unwired: 1 in]
            n156 = Bundle(w218, w251) -> (w246:cluster{dbl[], dbl[]})  [unwired: 1 in]
            n157 = Format Into String(format string="# Hx-Vx Mean Difference - %.4f  StdDev - %.4f\\r\\n# Slope - %.4f Intercept - %.4f", w217, w216, w215, w214) -> (resulting string=w191:string)  [unwired: 2 in, 1 out]
            n158 = Build Array (concatenate)(w209, w208, w207, "# SigGen GHz   dbmHc      dbmHx      dbmVc      dbmVx", w187, w188, w189, w190, w191) -> (w228:string[])
            n159 = Write to Text File(file (use dialog)=w241, text=w228, error in=w240) -> (refnum out=w239:refnum<file>, error out=w238:errorcluster)  [unwired: 1 in, 1 out]
            n160 = Close File(refnum=w239, error in=w238) -> (path=w235:path)  [unwired: 1 out]
            n161 = Build Array(w250, w249) -> (→"?":cluster{dbl[], dbl[]}[])
            n162 = Build Array(w248, w247, w245, w246) -> (→"RVP8 Bandwidth":cluster{dbl[], dbl[]}[])
            n163 = call "RF_Sig_Gen.vi"("Signal Generator Control"=T5 {"Frequency (GHz)"=2.809, "RF Power (dBm)"=-120.0, "RF ON/OFF"=FALSE}, "error in"=w231) -> ("Signal Generator Status"=w232:T7)  [unwired: 12 in, 1 out]
            n164 = Concatenate Strings("Data Directory", "/" ("string"), w206) -> (w236:string)
            n165 = String To Path(string=w236) -> (path=w234:path)
            n166 = local write "Signal Generator Status"(w232) -> ()
            n167 = Move(source path=w235, 10:w234) -> (3:→"Cal Output File":path)  [unwired: 3 in, 2 out]
          }
        }
        n168 = property on="Ready" class="Bool"("Visible"=w156) -> ()  [unwired: 2 in, 2 out]
        n169 = property on="RVP8 Bandwidth" class="XYGraph (strict)"("Visible"=w161) -> ()  [unwired: 2 in, 2 out]
        n170 = property class="XYGraph (strict)"("Visible"=w160) -> ()  [unwired: 2 in, 2 out]
        n171 = property on="Real Time XY" class="XYGraph (strict)"("Visible"=w159) -> ()  [unwired: 2 in, 2 out]
        n172 = local write "C-State"(w168) -> ()
      }
      frame #7 {
        # "Releasing the\nqueue stops\nthe consumer loop(s)."
        n173 = local write "C-State"(w299) -> ()
        n174 = Release Queue(queue=w298) -> ()  [unwired: 2 in, 3 out]
      }
    }
  }
  "Instructions" <- "rvp8 bandwidth measuring vi\n\nBasic operation:\u0000\u0000\n1 - configure ATE switches with the yellow 'Bandwidth Setup' button\u0000\u0000\n2 - measure the bandwidth with the red 'Calibrate' button\n3 - exit the program with the red 'Exit' button\n\nHints:\nWait for the green 'READY' light before clicking buttons\nClick appropriate blue buttons after making changes on 'Controls' tab\nCheck status tab before calibration" ("String")
